vi "construct.vi"(8 "error in (no error)":errorcluster, 9 "configuration name":string, 10 "load config file?":bool=TRUE, 11 "GenericPlugin in":refnum<class "TrajectoryAK101022Resonance.lvclass">) -> (0 "error out":errorcluster, 3 "GenericPlugin out":refnum<class "TrajectoryAK101022Resonance.lvclass">)   [LabVIEW 2010, in "TrajectoryAK101022Resonance.lvclass"]
uses:
  TrajectoryAK101022Resonance.lvclass
  TrajectoryMG100122GenericFPGA/TrajectoryMG100122GenericFPGA/TrajectoryMG100122GenericFPGA.lvclass
  FPGAWrapper/FPGAWrapperAK101022Resonance/FPGAWrapperAK101022Resonance/FPGAWrapperAK101022Resonance.lvclass
  FPGAWrapper/GenericFPGAWrapper/GenericFPGAWrapper/GenericFPGAWrapper.lvclass
  TrajectoryAK101022Resonance.lvclass/TrajectoryAK101022Resonance.ctl
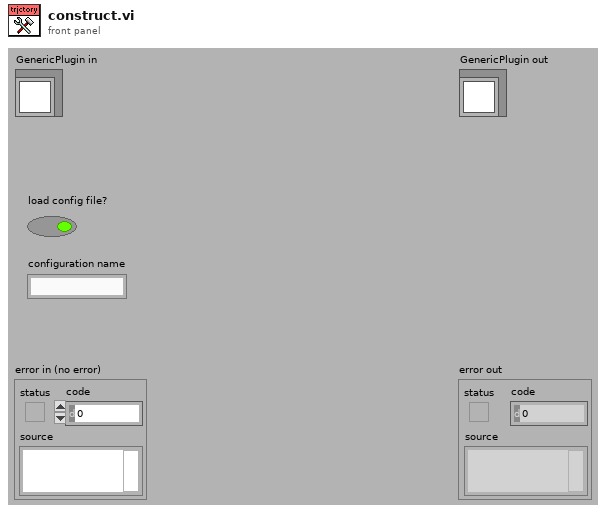
[diagram p1: front panel]
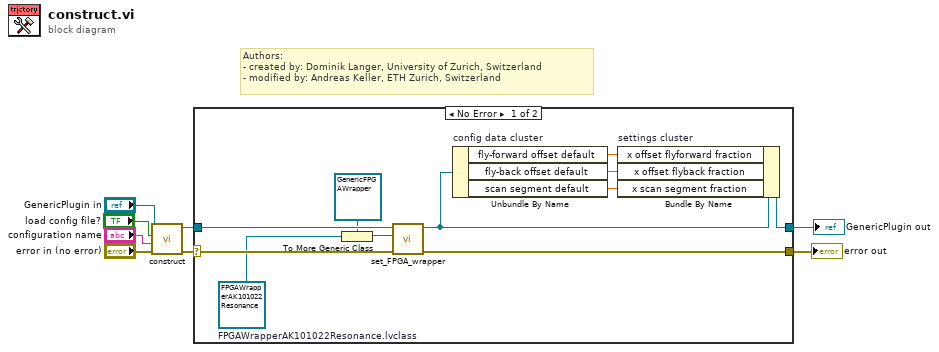
[diagram p0: block diagram]
diagram:
  # "Authors: \n- created by: Dominik Langer, University of Zurich, Switzerland\n- modified by: Andreas Keller, ETH Zurich, Switzerland"
  n1 = call-parent "construct.vi"("error in (no error)"="error in (no error)", "configuration name"="configuration name", "load config file?"="load config file?", "GenericPlugin in"="GenericPlugin in") -> ("error out"=w4:errorcluster, "GenericPlugin out"=w3:refnum<class "TrajectoryAK101022Resonance.lvclass">)  [unwired: 6 in]
  n2 = case shown="No Error" w4 {
    selector: w4 -> [w19 w20]
    tunnel: w3 -> [w18 w21]
    tunnel: [w17 w20] -> w2
    tunnel: [w10 w21] -> w1
    frame No Error {
      w9 = refnum<class "FPGAWrapperAK101022Resonance.lvclass"> refnum  # FPGAWrapperAK101022Resonance.lvclass
      n3 = To More Generic Class(target class=refnum<class "GenericFPGAWrapper.lvclass"> refnum ("GenericFPGAWrapper.lvclass"), reference=w9) -> (generic class reference=w15:refnum<class "GenericFPGAWrapper.lvclass">)
      n4 = call-dynamic "set_FPGA_wrapper.vi"("error in (no error)"=w19, "GenericFPGAWrapper.lvclass"=w15, "TrajectoryMG100122GenericFPGA in"=w18) -> ("error out"=w17:errorcluster, "TrajectoryMG100122GenericFPGA out"=w11:refnum<class "TrajectoryAK101022Resonance.lvclass">)  [unwired: 7 in]
      n5 = Unbundle By Name "config data cluster"(w11) -> ("fly-forward offset default"=w14:dbl, "fly-back offset default"=w13:dbl, "scan segment default"=w12:dbl)
      n6 = Bundle By Name "settings cluster"(cluster=w11, "x offset flyforward fraction"=w14, "x offset flyback fraction"=w13, "x scan segment fraction"=w12) -> (w10:refnum<class "TrajectoryAK101022Resonance.lvclass">)
    }
    frame Error {
    }
  }
  "error out" <- w2
  "GenericPlugin out" <- w1
